vi "Init.vi"(7 "User Type":refnum<class "User.lvclass">, 10 "Entity Manager":refnum<class "Entity Manager.lvclass">) -> (3 "User Provider out":refnum<class "User Provider.lvclass">)   [LabVIEW 2020, in "HTTP-Conditum.lvlib" / "User Provider.lvclass"]
uses:
  User Provider.lvclass
  <vilib>/IlluminatedG/IG Conditum/Conditum/Entity Manager/Entity Manager.lvclass
  User/User.lvclass
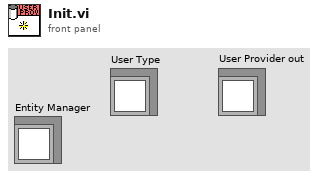
[diagram p1: front panel]
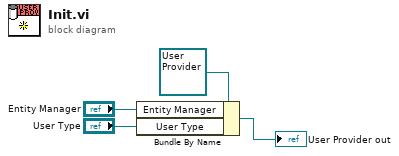
[diagram p0: block diagram]
diagram:
  n1 = Bundle By Name(cluster=refnum<class "User Provider.lvclass"> refnum ("User Provider in"), "Entity Manager"="Entity Manager", "User Type"="User Type") -> (→"User Provider out":refnum<class "User Provider.lvclass">)
